vi "ClimberSingleton.vi"(10 "Enum":enum16{"Get", "Set"}(ring), 11 "Climber.lvclass":refnum<class "Climber.lvclass">) -> (3 "Climber.lvclass":refnum<class "Climber.lvclass">)   [LabVIEW 2016, in "Climber.lvclass"]
uses:
  Climber.lvclass
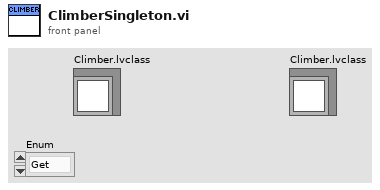
[diagram p1: front panel]
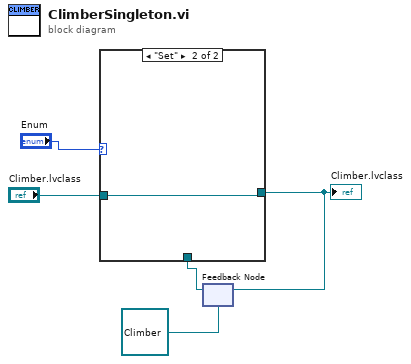
[diagram p0: block diagram]
diagram:
  n1 = feedback #1(refnum<class "Climber.lvclass"> refnum ("Climber.lvclass")) -> (w2:refnum<class "Climber.lvclass">)
  n2 = case shown="\"Set\"" "Enum" {
    tunnel: "Climber.lvclass" -> [_ w7]
    tunnel: w2 -> [w6 _]
    tunnel: [w6 w7] -> w1
    frame "Get", Default {
    }
    frame "Set" {
    }
  }
  "Climber.lvclass" <- w1
  n3 = feedback-in #1(w1) -> ()
